vi "Dynamic_call.vi"(8 "Error In":errorcluster, 11 "Limit":string="-5.1~-4.9") -> (0 "Error Out":errorcluster, 2 "TestResult":bool, 3 "TestData":string, 4 "ITEM":string, 5 "Limit":string="-5.1~-4.9")   [LabVIEW 2013]
uses:
  MainProgram/Control/Buffer.vi
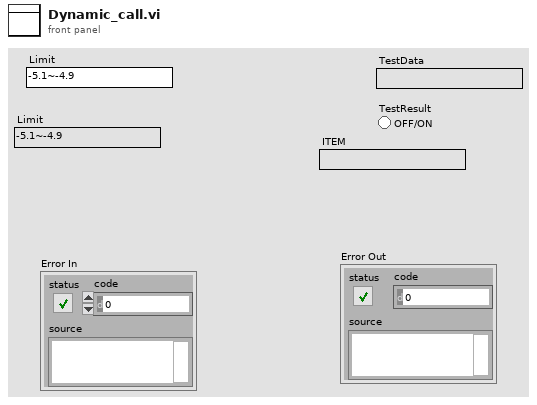
[diagram p1: front panel]
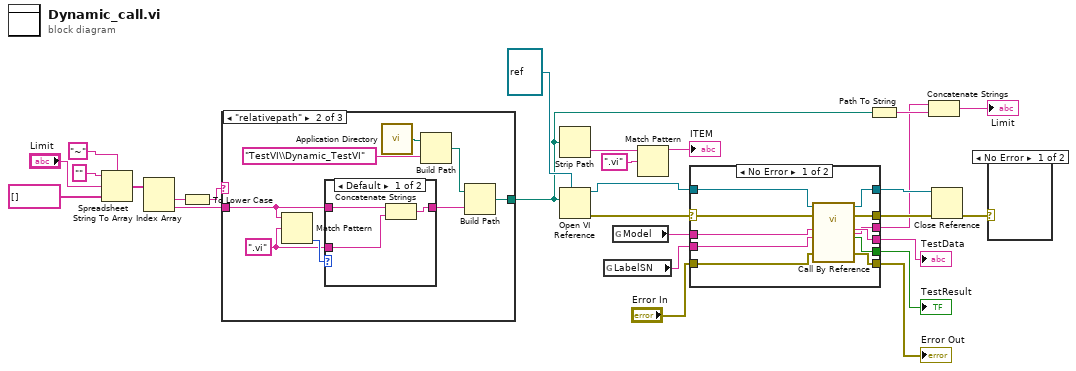
[diagram p0: block diagram]
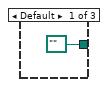
[diagram p2: hidden frame]
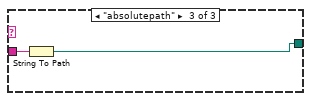
[diagram p4: hidden frame]
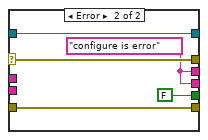
[diagram p6: hidden frame]
diagram:
  n1 = Spreadsheet String To Array(delimiter (Tab)="~", format string="", spreadsheet string="Limit", array type (2D Dbl)=string[] []) -> (array=w23:string[])
  n2 = Index Array(array=w23) -> (element #1=w7:string, element #2=w15:string)  [unwired: 2 in]
  n3 = To Lower Case(string=w7) -> (all lower case string=w6:string)
  n4 = case shown="\"relativepath\"" w6 {
    tunnel: w15 -> [_ w30 w42]
    tunnel: [path "" w33 w41] -> w5
    frame Default {
    }
    frame "relativepath" {
      w29 = ".vi" ("regular expression")
      n5 = Match Pattern(string=w30, regular expression=w29) -> (offset past match=w32:i32)  [unwired: 1 in, 3 out]
      n6 = case shown="Default" w32 {
        tunnel: [w38 w40] -> w31
        tunnel: w30 -> [w39 w40]
        tunnel: w29 -> [w37 _]
        frame Default {
          n7 = Concatenate Strings(w39, w37) -> (w38:string)
        }
        frame 0..9999 {
        }
      }
      n8 = call <vilib>:"Application Directory.vi"() -> ("Application Directory"=w36:path)
      n9 = Build Path(base path=w36, name or relative path="TestVI\\Dynamic_TestVI") -> (appended path=w34:path)
      n10 = Build Path(base path=w34, name or relative path=w31) -> (appended path=w33:path)
    }
    frame "absolutepath" {
      n11 = String To Path(string=w42) -> (path=w41:path)
    }
  }
  n12 = Strip Path(path=w5) -> (name=w9:string)  [unwired: 1 out]
  n13 = Open VI Reference(type specifier VI Refnum (for type only)=refnum<vi> refnum, vi path=w5) -> (vi reference=w13:refnum<vi>, error out=w1:errorcluster)  [unwired: 4 in]
  n14 = global read "Buffer.vi" "LabelSN"() -> (w17:string)
  n15 = global read "Buffer.vi" "Model"() -> (w19:string)
  n16 = Match Pattern(string=w9, regular expression=".vi") -> (before substring=→"ITEM":string)  [unwired: 1 in, 3 out]
  n17 = case shown="No Error" w1 {
    selector: w1 -> [w47 w55]
    tunnel: w13 -> [w53 w57]
    tunnel: [w52 FALSE ("Result")] -> w21
    tunnel: [w51 w57] -> w12
    tunnel: [w50 w55] -> w11
    tunnel: [w46 w54] -> w22
    tunnel: "Error In" -> [w49 w58]
    tunnel: [w48 w58] -> w20
    tunnel: [w45 w54] -> w3
    tunnel: w19 -> [w44 _]
    tunnel: w17 -> [w43 _]
    frame No Error {
      n18 = call-by-ref "?"(reference=w53, error in=w47, 8:"error in (no error)"=w49, "SN"=w43, "Model"=w44) -> (reference out=w51:refnum<vi>, error out=w50:errorcluster, 0:"error out"=w48:errorcluster, "Result"=w52:bool, "Data"=w46:string, "Limit"=w45:string)  [unwired: 5 in]
    }
    frame Error {
      w54 = "configure is error" ("Data")
    }
  }
  "TestResult" <- w21
  "TestData" <- w22
  "Error Out" <- w20
  n19 = Path To String(path=w5) -> (string=w4:string)
  n20 = Concatenate Strings(w3, w4) -> (→"Limit":string)
  n21 = Close Reference(reference=w12, error in (no error)=w11) -> (error out=w10:errorcluster)
  n22 = case shown="No Error" w10 {
    frame No Error {
    }
    frame Error {
    }
  }
